vi "Command History.vi"(1 "Data":string, 2 "Time":string) -> (0 "History":string)   [LabVIEW 2019, in "SubVIs.lvlib" / "Command VI.lvlib"]
uses:
  Command VI.lvlib
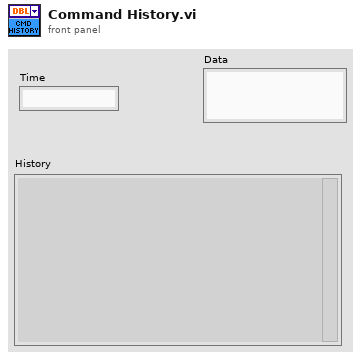
[diagram p1: front panel]
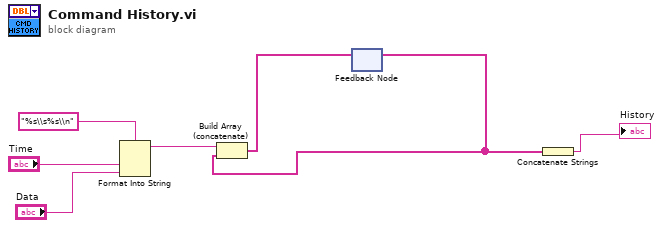
[diagram p0: block diagram]
diagram:
  n1 = Format Into String(format string="%s\\s%s\\n", "Time", "Data") -> (resulting string=w7:string)  [unwired: 2 in, 1 out]
  n2 = feedback #1() -> (w1:string[])  [unwired: 1 in]
  n3 = Build Array (concatenate) "Build Array"(w7, w1) -> (w2:string[])
  n4 = feedback-in #1(w2) -> ()
  n5 = Concatenate Strings(w1) -> (→"History":string)
